vi "Set Output State.vi"(8 "error in (no error)":cluster{"状态":bool, "代码":i32, "源":string} caption="错误输入（无错误）", 10 "输出状态":bool, 11 "蒸发冷却器":refnum<class "Evaporative Cooler.lvclass">) -> (0 "error out":cluster{"状态":bool, "代码":i32, "源":string} caption="错误输出", 3 "蒸发冷却器":refnum<class "Evaporative Cooler.lvclass">)   [LabVIEW 2013, in "Evaporative Cooler.lvlib" / "Evaporative Cooler.lvclass"]
doc: "子类中不应对该方法进行重写。如子类需要对该VI进行重写，则必须采用“调用父项”节点。"
uses:
  Evaporative Cooler.lvclass
  Evaporative Cooler.lvclass/Evaporative Cooler.ctl
  <vilib>/ActorFramework/Time-Delayed Send Message/Time-Delay Override Options.ctl
  <vilib>/ActorFramework/Message Enqueuer/Message Enqueuer.lvclass/Message Enqueuer.ctl
  Dual Fan/Run Fan Msg/Run Fan Msg.lvclass
  <vilib>/ActorFramework/Message Enqueuer/Enqueue.vi
  <vilib>/ActorFramework/Message Priority Queue/Priority Enqueue.vi
  Dual Fan/Halt Fan Msg/Halt Fan Msg.lvclass
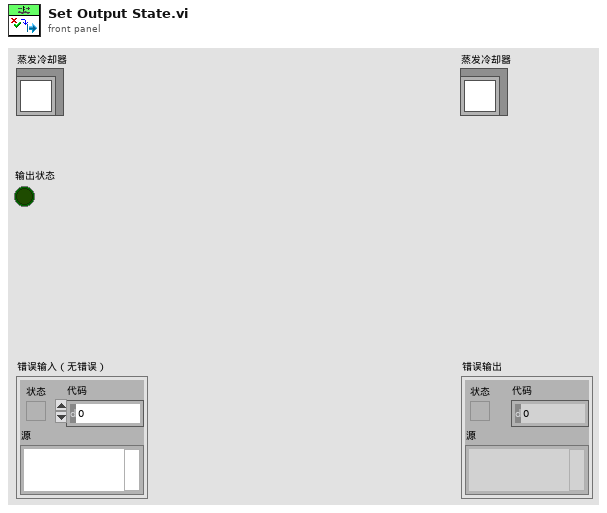
[diagram p1: front panel]
types:
  T1 = typedef "Time-Delay Override Options.ctl" = enum16{"Send next copy now", "Skip next scheduled copy", "Send next copy now and stop all further copies", "Stop all further copies"}
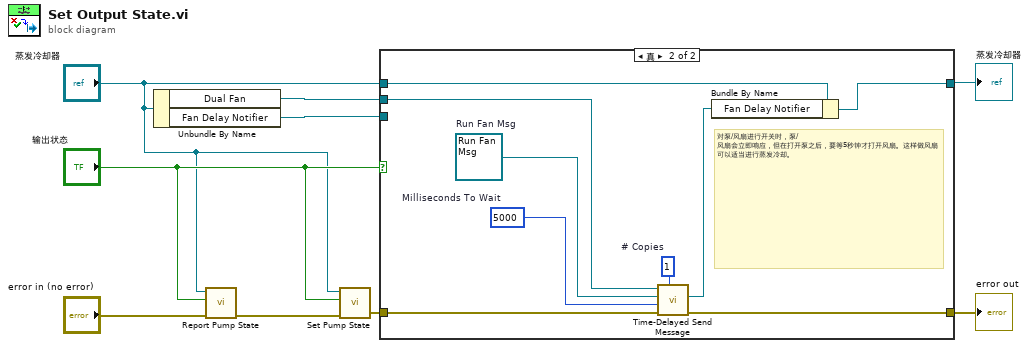
[diagram p0: block diagram]
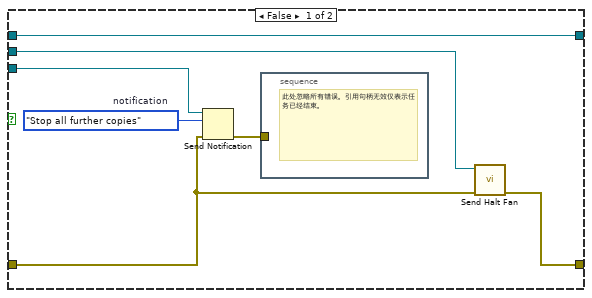
[diagram p2: hidden frame]
diagram:
  n1 = Unbundle By Name("蒸发冷却器") -> ("Dual Fan"=w9:refnum<class "Message Enqueuer.lvclass">, "Fan Delay Notifier"=w6:refnum<notifier>)
  n2 = call "Report Pump State.vi"("error in (no error)"="error in (no error)", "泵状态"="输出状态", "蒸发冷却器输入"="蒸发冷却器") -> ("error out"=w3:cluster{"状态":bool, "代码":i32, "源":string})  [unwired: 8 in]
  n3 = call-dynamic "Set Pump State.vi"("error in (no error)"=w3, "泵状态"="输出状态", "蒸发冷却器输入"="蒸发冷却器") -> ("error out"=w4:cluster{"状态":bool, "代码":i32, "源":string})  [unwired: 8 in]
  n4 = case shown="真" "输出状态" {
    tunnel: w4 -> [w10 w25]
    tunnel: w9 -> [w15 w19]
    tunnel: [w16 w24] -> w8
    tunnel: "蒸发冷却器" -> [w14 w22]
    tunnel: [w14 w21] -> w7
    tunnel: w6 -> [w13 _]
    frame False {
      w12 = Time-Delay_Override_Options."Stop all further copies"  # notification
      n5 = Send Notification(notification=w12, notifier=w13, error in (no error)=w10) -> (error out=w11:errorcluster)  [unwired: 1 out]
      n6 = stacked-sequence {
        tunnel: w11 -> [_]
        frame #0 {
          # "此处忽略所有错误。引用句柄无效仅表示任务已经结束。"
        }
      }
      n7 = call "Send Halt Fan.vi"("error in (no error)"=w10, "消息待入队列"=w15) -> ("error out"=w16:cluster{"状态":bool, "代码":i32, "源":string})  [unwired: 9 in]
    }
    frame True {
      w17 = 5000  # Milliseconds To Wait
      w18 = refnum<class "Run Fan Msg.lvclass"> refnum  # Run Fan Msg
      w23 = u32 1  # # Copies
      # "对泵/风扇进行开关时，泵/风扇会立即响应，但在打开泵之后，要等5秒钟才打开风扇。这样做风扇可以适当进行蒸发冷却。"
      n8 = call <vilib>:"Time-Delayed Send Message.vi"("# Copies (0 = infinite repeat)"=w23, "error in (no error)"=w25, "Milliseconds To Wait"=w17, "Message"=w18, "Message Enqueuer"=w19) -> ("error out"=w24:errorcluster, "Delivery Notifier"=w20:refnum<notifier>)  [unwired: 5 in]
      n9 = Bundle By Name(cluster=w22, "Fan Delay Notifier"=w20) -> (w21:refnum<class "Evaporative Cooler.lvclass">)
    }
  }
  "error out" <- w8
  "蒸发冷却器" <- w7
